vi "Teleop.vi"(10 "Match Info":T2={"Autonomous Elapsed Seconds"=0.0, "TeleOp Elapsed Seconds"=0.0, "Disabled Elapsed Seconds"=0.0, "Visited Autonomous"=FALSE, "Visited TeleOp"=FALSE, "Visited Disabled"=FALSE, "Autonomous Settings"={"Autonomous Style"=enum."Independent", "VI Refnum"=refnum}}, 11 "Call Context":T3) -> ()   [LabVIEW 2013]
doc: "This VI is called for each TeleOp packet received from the DS where the robot is not disabled. It is often used to read from the joysticks and update I/O or to update setpoints for timed control loops. It should complete and return within 20 milliseconds or it may miss DS packets."
uses:
  <vilib>/Rock Robotics/WPI/DriverStation/WPI_DriverStationDerivedRobotMode.ctl
  <vilib>/Rock Robotics/WPI/DriverStation/WPI_DriverStationMatch Info.ctl
  Robot Global Data.vi
  <vilib>/Rock Robotics/WPI/RobotDrive/WPI_RobotDriveArcadeDrive_Standard(NoSaturation).vi
  <vilib>/Rock Robotics/WPI/Joystick/WPI_JoystickGetSetRefNum.vi
  <vilib>/Rock Robotics/WPI/RobotDrive/WPI_RobotDriveGetSetRefNum.vi
panel:
  in  "Triggertime":u32=800
  in  "Pausetime":u32=1200
  in  "Start Time":u32=1500
  out "State":T1(ring)
  in  "Trigger Speed":dbl=0.5
  in  "ShooterSpeed":dbl=0.4
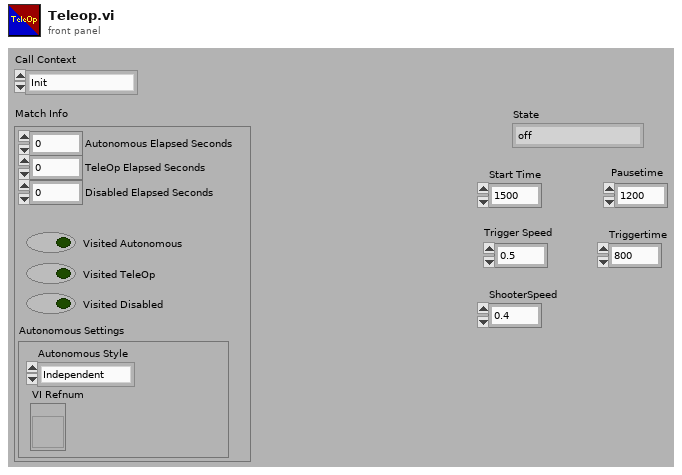
[diagram p1: front panel]
types:
  T1 = enum16{"off", "Start Shooter", "trigger fwd", "trigger bkwd"}
  T2 = typedef "WPI_DriverStationMatch Info.ctl" = cluster{"Autonomous Elapsed Seconds":dbl, "TeleOp Elapsed Seconds":dbl, "Disabled Elapsed Seconds":dbl, "Visited Autonomous":bool, "Visited TeleOp":bool, "Visited Disabled":bool, "Autonomous Settings":cluster{"Autonomous Style":enum16{"Iterative", "Independent"}, "VI Refnum":refnum<vi>}}
  T3 = typedef "WPI_DriverStationDerivedRobotMode.ctl" = enum16{"Init", "Execute", "Stop"}
  T4 = typedef "WPI_JoystickDevRef.ctl" = cluster{"Device":T5}
  T5 = typedef "WPI_JoystickDeviceEnum.ctl" = enum16{"USB 1", "USB 2", "USB 3", "USB 4", "Kinect 1", "Kinect 2"}
  T6 = typedef "WPI_JoystickButtonState.ctl" = cluster{"Button 1":bool, "Button 2":bool, "Button 3":bool, "Button 4":bool, "Button 5":bool, "Button 6":bool, "Button 7":bool, "Button 8":bool, "Button 9":bool, "Button 10":bool, "Button 11":bool, "Button 12":bool}
  T7 = cluster{"axis 1 (x)":dbl, "axis 2 (y)":dbl, "axis 3 (throttle)":dbl, "axis 4":dbl, "axis 5":dbl, "axis 6":dbl}
  T8 = typedef "WPI_DigitalInputDevRef.ctl" = cluster{"DevStatus":errorcluster, "DIO Channel":T9, "Digital Module":T10}
  T9 = typedef "FPGA_DIOChannel.ctl" = enum8{"DIO 1", "DIO 2", "DIO 3", "DIO 4", "DIO 5", "DIO 6", "DIO 7", "DIO 8", "DIO 9", "DIO 10", "DIO 11", "DIO 12", "DIO 13", "DIO 14", "Invalid"}
  T10 = typedef "FPGA_TypedefDigitalModule.ctl" = enum16{"Digital Module 1", "Digital Module 2"}
  T11 = enum16{"off", "Start Shooter", "trigger fwd", "trigger bkwd", "Pause"}
  T12 = typedef "WPI_RobotDriveDevRef.ctl" = cluster{"DevStatus":errorcluster, "Motors[]":T13[], "Square Inputs":bool, "Max Output":dbl, "Isochronous":bool}
  T13 = typedef "WPI_MotorControlDeviceRef.ctl" = cluster{"DeviceStatus":errorcluster, "Type":enum16{"PWM", "CAN"}, "PWM":cluster{"Digital Module":T10, "PWM Channel":T14, "DeadBand":T15}, "CAN":cluster{"Device Number":u8, "Control Mode":T16, "Semaphore":T17, "Max Vout":dbl}, "Invert":bool, "TransformRef":T18, "InvTransformRef":T18}
  T14 = typedef "FPGA_DIOPWMChannel.ctl" = enum8{"PWM 1", "PWM 2", "PWM 3", "PWM 4", "PWM 5", "PWM 6", "PWM 7", "PWM 8", "PWM 9", "PWM 10", "Invalid"}
  T15 = typedef "WPI_PWMDeadband.ctl" = cluster{"Name":string, "maxPositivePwm":i32, "minPositivePwm":i32, "centerPwm":i32, "maxNegativePwm":i32, "minNegativePwm":i32, "angularRange":u16}
  T16 = typedef "WPI_CANJaguar_ControlMode.ctl" = enum8{"Percent VBus", "Current", "Speed", "Position", "Voltage"}
  T17 = typedef "Semaphore RefNum" = refnum<k1>
  T18 = typedef "WPI_PWMTransform_ConPane.ctl" = refnum<vi>
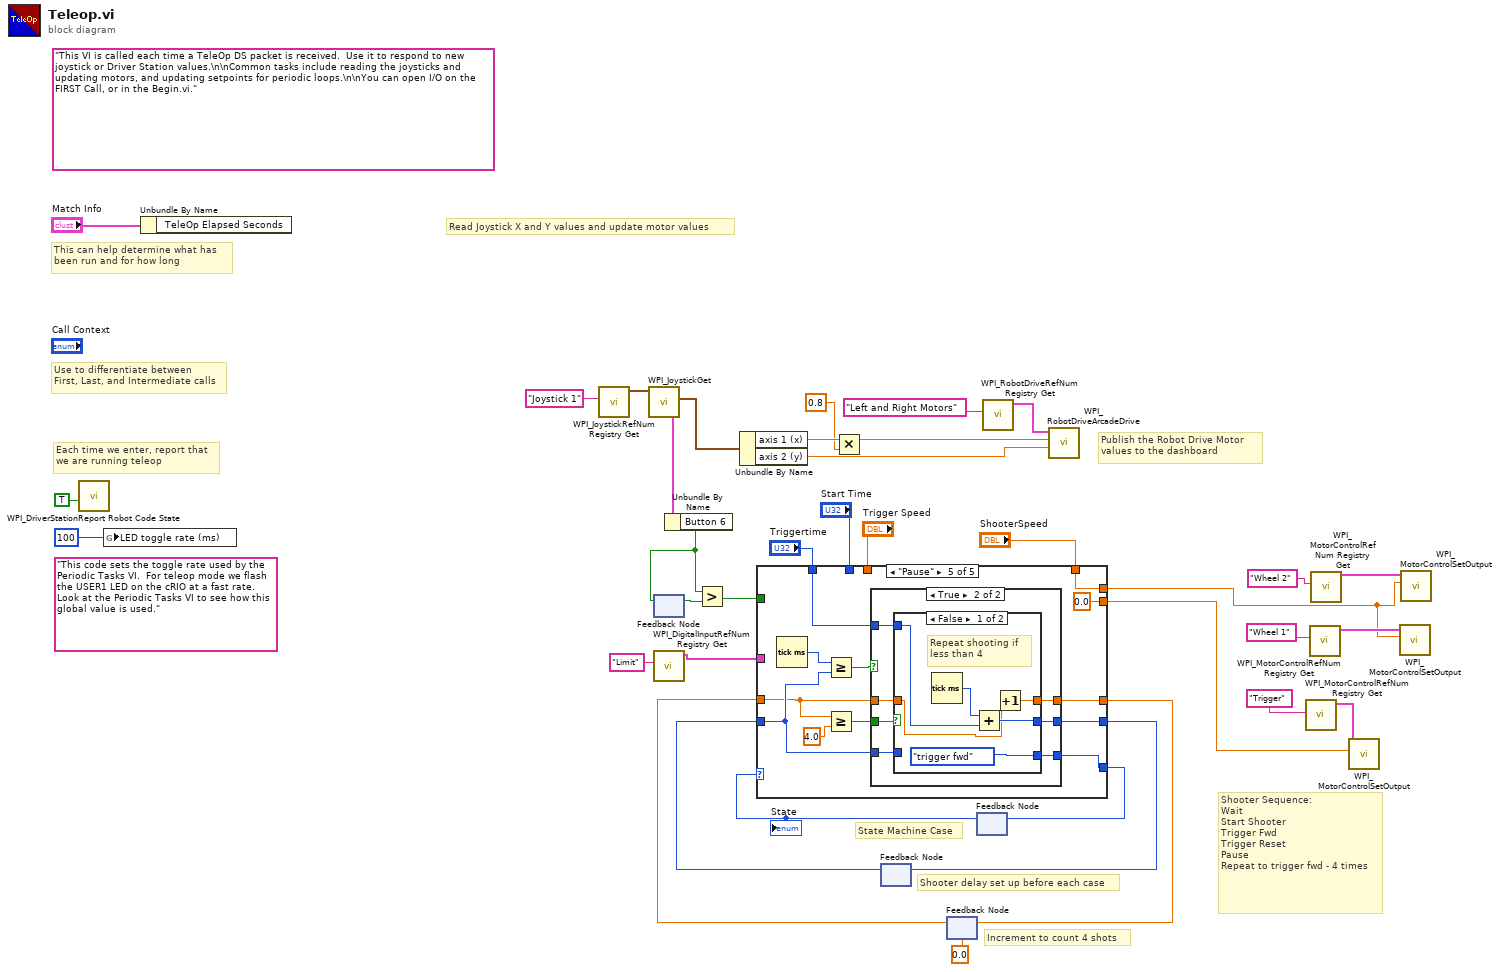
[diagram p0: block diagram]
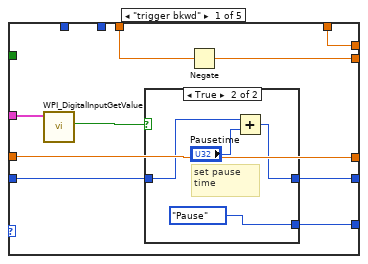
[diagram p2: hidden frame]
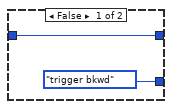
[diagram p3: hidden frame]
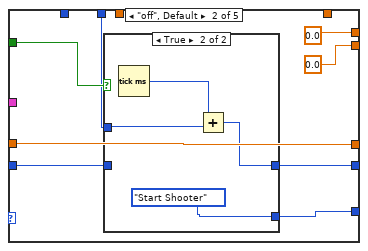
[diagram p4: hidden frame]
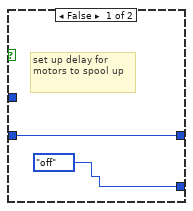
[diagram p5: hidden frame]
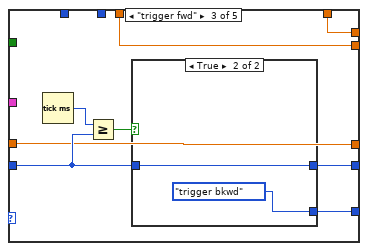
[diagram p6: hidden frame]
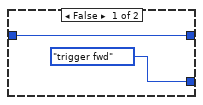
[diagram p7: hidden frame]
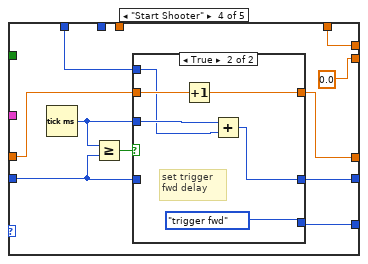
[diagram p8: hidden frame]
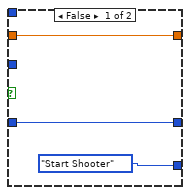
[diagram p9: hidden frame]
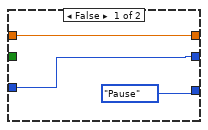
[diagram p10: hidden frame]
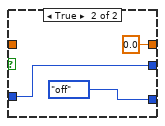
[diagram p11: hidden frame]
diagram:
  (unwired) "This code sets the toggle rate used by the Periodic Tasks VI.  For teleop mode we flash the USER1 LED on the cRIO at a fast rate.  Look at the Periodic Tasks VI to see how this global value is used."
  (unwired) "This VI is called each time a TeleOp DS packet is received.  Use it to respond to new joystick or Driver Station values.\n\nCommon tasks include reading the joysticks and updating motors, and updating setpoints for periodic loops.\n\nYou can open I/O on the FIRST Call, or in the Begin.vi."
  # "Shooter Sequence:\nWait\nStart Shooter \nTrigger Fwd\nTrigger Reset\nPause\nRepeat to trigger fwd - 4 times"
  # "Increment to count 4 shots"
  # "State Machine Case"
  # "Shooter delay set up before each case"
  # "Publish the Robot Drive Motor\nvalues to the dashboard"
  # "Each time we enter, report that\nwe are running teleop"
  # "Use to differentiate between\nFirst, Last, and Intermediate calls"
  # "This can help determine what has\nbeen run and for how long"
  # "Read Joystick X and Y values and update motor values"
  n1 = call <vilib>:"WPI_DriverStationReport Robot Code State.vi"("TeleOp"=TRUE ("Autonomous")) -> ()  [unwired: 10 in, 1 out]
  n2 = global write "Robot Global Data.vi" "LED toggle rate (ms)"(u32 100 ("LED ms toggle rate")) -> ()
  n3 = Unbundle By Name("Match Info") -> ()  [unwired: 1 out]
  n4 = call <vilib>:"WPI_JoystickRefNum Registry Get.vi"("refnum name"="Joystick 1") -> ("JoystickDevRef"=w31:T4)  [unwired: 1 in, 9 out]
  n5 = call <vilib>:"WPI_JoystickGet.vi"("JoystickDevRef"=w31) -> ("Buttons"=w27:T6, "Axes"=w28:T7)  [unwired: 1 in, 4 out]
  n6 = feedback #1() -> (w15:bool)  [unwired: 1 in]
  n7 = call <vilib>:"WPI_DigitalInputRefNum Registry Get.vi"("refnum name"="Limit") -> ("DigitalInputDevRef"=w19:T8)  [unwired: 9 in, 1 out]
  n8 = Unbundle By Name(w27) -> ("Button 6"=w16:bool)
  n9 = feedback-in #1(w16) -> ()
  n10 = Greater?(x=w16, y=w15) -> (0:w17:bool)
  n11 = Unbundle By Name(w28) -> ("axis 1 (x)"=w34:dbl, "axis 2 (y)"=w33:dbl)
  n12 = Multiply(x=w34, y=0.8 ("axis 1 (x)")) -> (x*y=w2:dbl)
  n13 = feedback #2() -> (w11:u32)  [unwired: 1 in]
  n14 = feedback #3(0.0) -> (w6:dbl)
  n15 = feedback #4() -> (w8:T11)  [unwired: 1 in]
  "State" <- w8
  n16 = case shown="\"Pause\"" w8 {
    tunnel: [w45 0.0 w74 w87 w108] -> w14
    tunnel: [w41 w55 w71 w84 w109] -> w18
    tunnel: w19 -> [w46 _ _ _ _]
    tunnel: w17 -> [_ w58 _ _ _]
    tunnel: [w43 0.0 w73 0.0 0.0 ("Trigger Speed")] -> w13
    tunnel: [w39 w56 w70 w82 w106] -> w12
    tunnel: w11 -> [w40 w57 w69 w83 w103]
    tunnel: "ShooterSpeed" -> [w45 _ w74 w87 w108]
    tunnel: "Trigger Speed" -> [w44 _ w73 _ _]
    tunnel: [w38 w54 w67 w81 w100] -> w7
    tunnel: w6 -> [w38 w54 w67 w80 w99]
    tunnel: "Start Time" -> [_ w53 _ _ _]
    tunnel: "Triggertime" -> [_ _ _ w79 w98]
    frame "trigger bkwd" {
      n17 = call <vilib>:"WPI_DigitalInputGetValue.vi"("DigitalInputDevRef"=w46) -> ("Value"=w42:bool)  [unwired: 8 in, 2 out]
      n18 = case shown="True" w42 {
        tunnel: [T11."trigger bkwd" T11."Pause"] -> w41
        tunnel: [w48 w49] -> w39
        tunnel: w40 -> [w48 w50]
        frame False {
        }
        frame True {
          # "set pause time"
          n19 = Add(x=w50, y="Pausetime") -> (x+y=w49:u32)
        }
      }
      n20 = Negate(x=w44) -> (-x=w43:dbl)
    }
    frame "off", Default {
      n21 = case shown="True" w58 {
        tunnel: w57 -> [w62 _]
        tunnel: [w62 w65] -> w56
        tunnel: [T11."off" T11."Start Shooter"] -> w55
        tunnel: w53 -> [_ w63]
        frame False {
          # "set up delay for motors to spool up"
        }
        frame True {
          n22 = Tick Count (ms)() -> (millisecond timer value=w66:u32)
          n23 = Add(x=w66, y=w63) -> (x+y=w65:u32)
        }
      }
    }
    frame "trigger fwd" {
      n24 = Tick Count (ms)() -> (millisecond timer value=w68:u32)
      n25 = Greater Or Equal?(x=w68, y=w69) -> (x >= y?=w72:bool)
      n26 = case shown="True" w72 {
        tunnel: [T11."trigger fwd" T11."trigger bkwd"] -> w71
        tunnel: [w76 w78] -> w70
        tunnel: w69 -> [w76 w78]
        frame False {
        }
        frame True {
        }
      }
    }
    frame "Start Shooter" {
      n27 = Tick Count (ms)() -> (millisecond timer value=w85:u32)
      n28 = Greater Or Equal?(x=w85, y=w83) -> (x >= y?=w86:bool)
      n29 = case shown="True" w86 {
        tunnel: w85 -> [_ w97]
        tunnel: [T11."Start Shooter" T11."trigger fwd"] -> w84
        tunnel: w83 -> [w91 _]
        tunnel: [w91 w96] -> w82
        tunnel: [w90 w95] -> w81
        tunnel: w80 -> [w90 w94]
        tunnel: w79 -> [_ w92]
        frame False {
        }
        frame True {
          # "set trigger fwd delay"
          n30 = Increment(x=w94) -> (x+1=w95:dbl)
          n31 = Add(x=w97, y=w92) -> (x+y=w96:u32)
        }
      }
    }
    frame "Pause" {
      n32 = Tick Count (ms)() -> (millisecond timer value=w104:u32)
      n33 = Greater Or Equal?(x=w104, y=w103) -> (x >= y?=w102:bool)
      n34 = Greater Or Equal?(x=w99, y=4.0) -> (x >= y?=w101:bool)
      n35 = case shown="True" w102 {
        tunnel: [T11."Pause" w119] -> w109
        tunnel: [w111 w118] -> w106
        tunnel: w98 -> [_ w117]
        tunnel: w103 -> [w111 w116]
        tunnel: w101 -> [_ w115]
        tunnel: [w110 w114] -> w100
        tunnel: w99 -> [w110 w113]
        frame False {
        }
        frame True {
          n36 = case shown="False" w115 {
            tunnel: [w123 w128] -> w118
            tunnel: [T11."trigger fwd" T11."off"] -> w119
            tunnel: w117 -> [w124 _]
            tunnel: w116 -> [_ w128]
            tunnel: [w120 0.0] -> w114
            tunnel: w113 -> [w121 _]
            frame False {
              # "Repeat shooting if less than 4"
              n37 = Tick Count (ms)() -> (millisecond timer value=w122:u32)
              n38 = Add(x=w122, y=w124) -> (x+y=w123:u32)
              n39 = Increment(x=w121) -> (x+1=w120:dbl)
            }
            frame True {
            }
          }
        }
      }
    }
  }
  n40 = feedback-in #2(w12) -> ()
  n41 = feedback-in #3(w7) -> ()
  n42 = feedback-in #4(w18) -> ()
  n43 = call <vilib>:"WPI_RobotDriveRefNum Registry Get.vi"("refnum name"="Left and Right Motors") -> ("RobotDriveDevRef"=w35:T12)  [unwired: 1 in, 9 out]
  n44 = call-poly <vilib>:"WPI_RobotDriveArcadeDrive.vi"("Y axis value"=w33, "X axis value"=w2, "RobotDriveDevRef"=w35) -> ()  [unwired: 6 in, 3 out]
  n45 = call <vilib>:"WPI_MotorControlRefNum Registry Get.vi"("refnum name"="Trigger") -> ("MotorControlDevRef"=w23:T13)  [unwired: 9 in, 1 out]
  n46 = call <vilib>:"WPI_MotorControlRefNum Registry Get.vi"("refnum name"="Wheel 1") -> ("MotorControlDevRef"=w26:T13)  [unwired: 9 in, 1 out]
  n47 = call <vilib>:"WPI_MotorControlRefNum Registry Get.vi"("refnum name"="Wheel 2") -> ("MotorControlDevRef"=w21:T13)  [unwired: 9 in, 1 out]
  n48 = call <vilib>:"WPI_MotorControlSetOutput.vi"("Output"=w13, "MotorControlDevRef"=w23) -> ()  [unwired: 7 in, 3 out]
  n49 = call <vilib>:"WPI_MotorControlSetOutput.vi"("Output"=w14, "MotorControlDevRef"=w26) -> ()  [unwired: 7 in, 3 out]
  n50 = call <vilib>:"WPI_MotorControlSetOutput.vi"("Output"=w14, "MotorControlDevRef"=w21) -> ()  [unwired: 7 in, 3 out]
